vi "DataReplay.vi"() -> ()   [LabVIEW 2018]
uses:
  <vilib>/Waveform/WDTFileIO.llb/Read Waveform from File.vi
  <vilib>/measure/maspectr.llb/FFT Spectrum (Mag-Phase) for N Chan.vi
  <vilib>/Analysis/3filter.llb/Zero Phase Filter (DBL).vi
  <vilib>/Analysis/baseanly.llb/Inverse f Filter (DBL).vi
  <vilib>/Analysis/3filter.llb/FIR Windowed Filter (DBL).vi
  <vilib>/Analysis/NI_AALBase.lvlib
  <vilib>/measure/NI_MAPro.lvlib
panel:
  in  "CH2 历史数据 2":u32(ring) items=["矩形"=0, "Hanning"=1, "Hamming"=2, "Blackman"=5, "Flat Top"=6]
  out "第一次波形":bool=TRUE
  in  "滤波器类型":enum32{"零相位滤波器", "反幂律滤波器", "FIR滤波器", "中值滤波器"}(ring)
  in  "CH2 历史数据":u16(ring) items=["2021-07-14-11-34-43.csv"]
  in  "数据重置":bool
  in  "停止":bool
  in  "CH1 历史数据":u16(ring) items=["2021-07-14-11-34-43.csv"]
  out "频谱图":cluster{"f0":dbl, "df":dbl, "magnitude":dbl[]}[](graph)
  out "滤波":dynamicdata(graph)
  out "原波形":dynamicdata(graph)
  # "原波形"
  # "数据选择"
  # "滤波"
  # "频谱图"
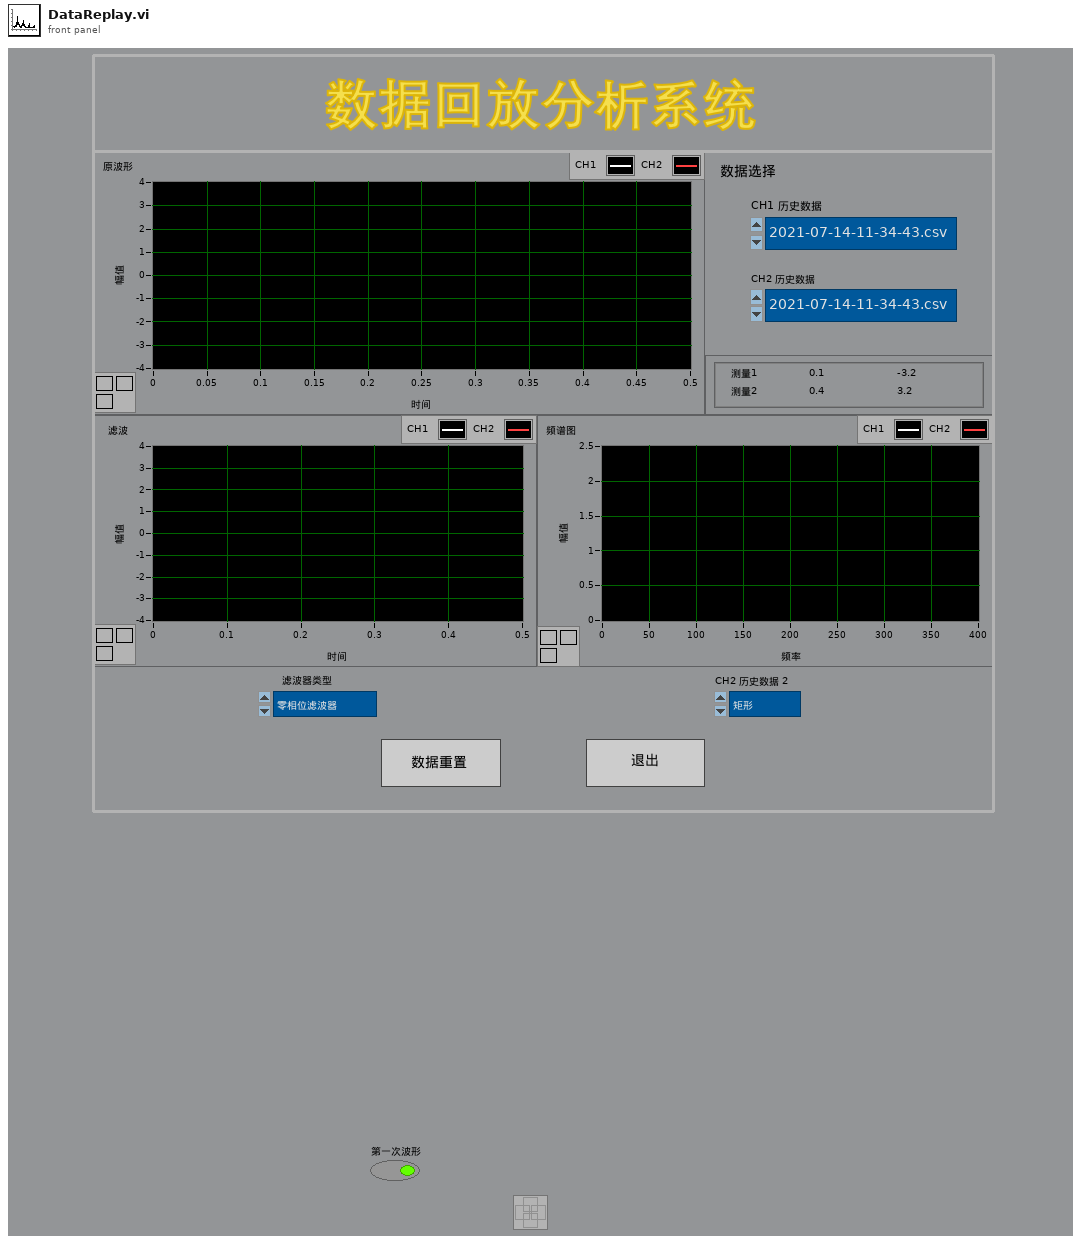
[diagram p1: front panel]
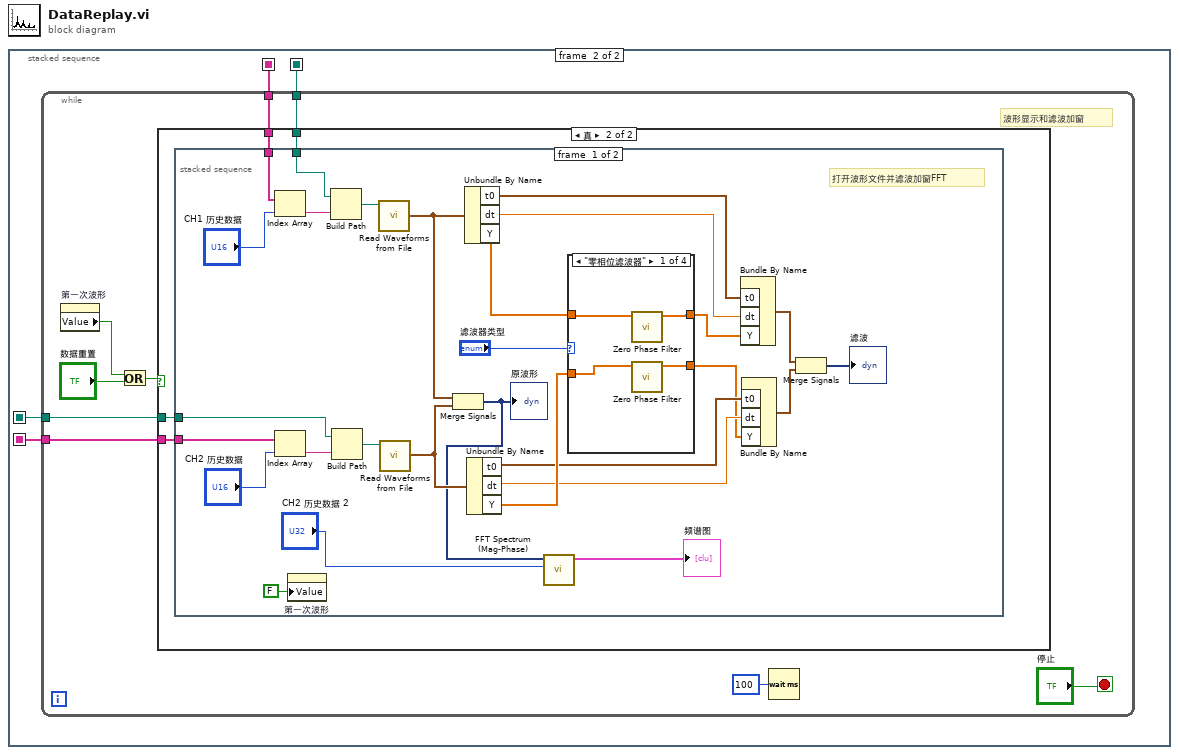
[diagram p0: block diagram]
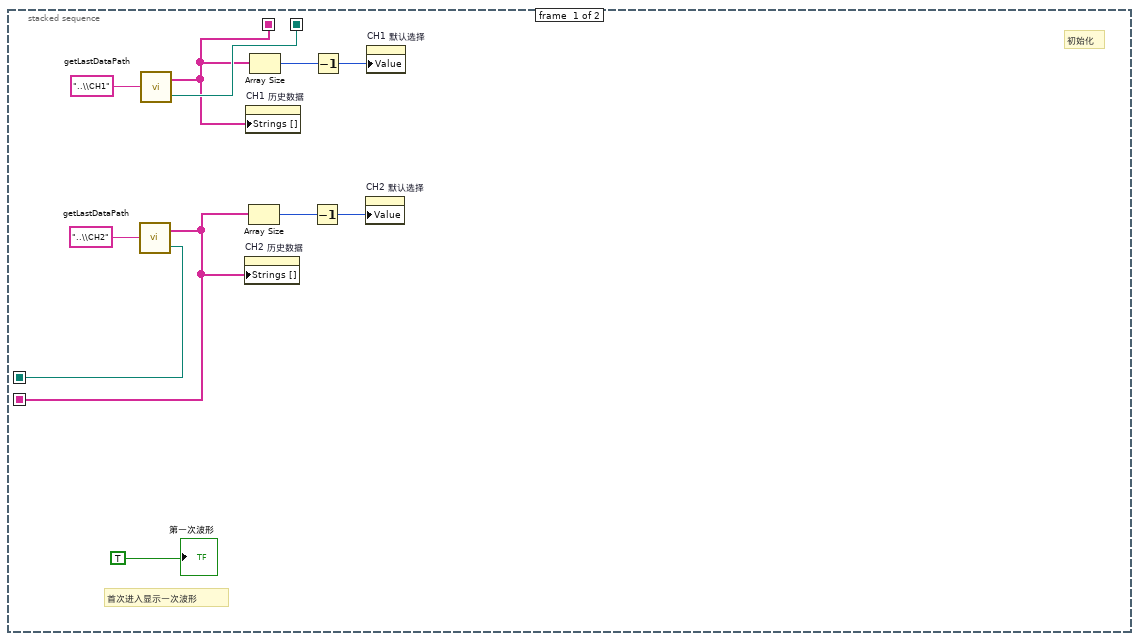
[diagram p2: hidden frame]
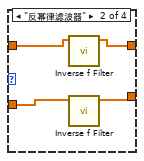
[diagram p4: hidden frame]
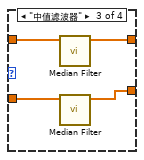
[diagram p5: hidden frame]
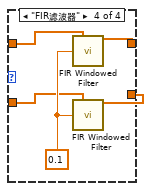
[diagram p6: hidden frame]
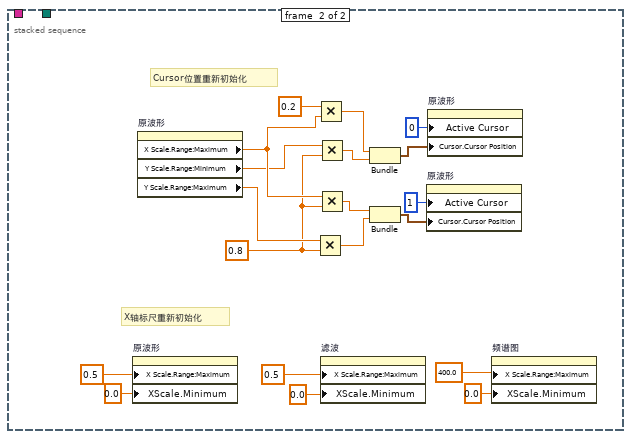
[diagram p7: hidden frame]
diagram:
  n1 = stacked-sequence {
    seq-local: [w8 _] -> [_ w15]
    seq-local: [w7 _] -> [_ w14]
    seq-local: [w2 _] -> [_ w12]
    seq-local: [w3 _] -> [_ w13]
    frame #0 {
      # "初始化"
      # "首次进入显示一次波形"
      n2 = call "getLastDataPath.vi"("文件夹输入"="..\\CH2" ("名称或相对路径")) -> ("数据文件名数组"=w2:string[], "文件夹路径"=w3:path)
      n3 = call "getLastDataPath.vi"("文件夹输入"="..\\CH1" ("名称或相对路径")) -> ("数据文件名数组"=w7:string[], "文件夹路径"=w8:path)
      n4 = property on="CH2 历史数据" class="Ring (严格)"("Strings []"=w2) -> ()  [unwired: 2 in, 2 out]
      n5 = property on="CH1 历史数据" class="Ring (严格)"("Strings []"=w7) -> ()  [unwired: 2 in, 2 out]
      n6 = Array Size(array=w2) -> (size(s)=w6:i32)
      n7 = Array Size(array=w7) -> (size(s)=w11:i32)
      n8 = Decrement(x=w6) -> (x-1=w5:i32)
      n9 = Decrement(x=w11) -> (x-1=w10:i32)
      n10 = property on="CH2 默认选择" class="Ring (严格)"("Value"=w5) -> ()  [unwired: 2 in, 2 out]
      n11 = property on="CH1 默认选择" class="Ring (严格)"("Value"=w10) -> ()  [unwired: 2 in, 2 out]
      "第一次波形" <- TRUE
    }
    frame #1 {
      n12 = while {
        tunnel: w15 -> [w22]
        tunnel: w14 -> [w21]
        tunnel: w13 -> [w20]
        tunnel: w12 -> [w19]
        stop <- "停止" stop-if-true
        # "波形显示和滤波加窗"
        n13 = property on="第一次波形" class="Bool (严格)"() -> ("Value"=w16:bool)  [unwired: 2 in, 2 out]
        n14 = Or(x=w16, y="数据重置") -> (x .or. y?=w17:bool)
        n15 = case shown="真" w17 {
          tunnel: w22 -> [_ w28]
          tunnel: w21 -> [_ w27]
          tunnel: w20 -> [_ w26]
          tunnel: w19 -> [_ w25]
          frame False {
          }
          frame True {
            n16 = stacked-sequence {
              tunnel: w28 -> [w53 _]
              tunnel: w27 -> [w52 _]
              tunnel: w26 -> [w48 _]
              tunnel: w25 -> [w47 _]
              frame #0 {
                # "打开波形文件并滤波加窗FFT"
                n17 = Index Array(array=w52, index="CH1 历史数据") -> (element=w55:string)
                n18 = Index Array(array=w47, index="CH2 历史数据") -> (element=w50:string)
                n19 = property on="第一次波形" class="Bool (严格)"("Value"=FALSE ("第一次波形")) -> ()  [unwired: 2 in, 2 out]
                n20 = Build Path(base path=w53, name or relative path=w55) -> (appended path=w54:path)
                n21 = Build Path(base path=w48, name or relative path=w50) -> (appended path=w49:path)
                n22 = call-poly <vilib>:"Read Waveforms from File.vi"("file path (dialog if empty)"=w54) -> ("first waveform in record"=w33:waveform(dbl))  [unwired: 5 in, 3 out]
                n23 = call-poly <vilib>:"Read Waveforms from File.vi"("file path (dialog if empty)"=w49) -> ("first waveform in record"=w32:waveform(dbl))  [unwired: 5 in, 3 out]
                n24 = Merge Signals(w33, w32) -> (w31:dynamicdata)
                "原波形" <- w31
                n25 = Unbundle By Name(w33) -> ("t0"=w42:timestamp, "dt"=w41:dbl, "Y"=w44:dbl[])
                n26 = Unbundle By Name(w32) -> ("t0"=w39:timestamp, "dt"=w38:dbl, "Y"=w43:dbl[])
                n27 = call-poly <vilib>:"FFT Spectrum (Mag-Phase).vi"("window"="CH2 历史数据 2", "time signals"=w31) -> ("magnitudes"=→"频谱图":cluster{"f0":dbl, "df":dbl, "magnitude":dbl[]}[])  [unwired: 5 in, 4 out]
                n28 = case shown="\"零相位滤波器\"" "滤波器类型" {
                  tunnel: w43 -> [w60 w64 w68 w72]
                  tunnel: [w59 w63 w67 w70] -> w40
                  tunnel: [w58 w62 w66 w71] -> w37
                  tunnel: w44 -> [w57 w61 w65 w69]
                  frame "零相位滤波器" {
                    n29 = call-poly <vilib>:"Zero Phase Filter.vi"("X"=w57) -> ("Filtered X"=w59:dbl[])  [unwired: 9 in, 1 out]
                    n30 = call-poly <vilib>:"Zero Phase Filter.vi"("X"=w60) -> ("Filtered X"=w58:dbl[])  [unwired: 9 in, 1 out]
                  }
                  frame "反幂律滤波器" {
                    n31 = call-poly <vilib>:"Inverse f Filter.vi"("X"=w61) -> ("Filtered X"=w63:dbl[])  [unwired: 6 in, 4 out]
                    n32 = call-poly <vilib>:"Inverse f Filter.vi"("X"=w64) -> ("Filtered X"=w62:dbl[])  [unwired: 6 in, 4 out]
                  }
                  frame "中值滤波器" {
                    n33 = call <vilib>:"Median Filter.vi"("X"=w65) -> ("Filtered X"=w67:dbl[])  [unwired: 9 in, 1 out]
                    n34 = call <vilib>:"Median Filter.vi"("X"=w68) -> ("Filtered X"=w66:dbl[])  [unwired: 9 in, 1 out]
                  }
                  frame "FIR滤波器" {
                    w73 = 0.1
                    n35 = call-poly <vilib>:"FIR Windowed Filter.vi"("X"=w69, "low cutoff freq: fl"=w73) -> ("Filtered X"=w70:dbl[])  [unwired: 12 in, 1 out]
                    n36 = call-poly <vilib>:"FIR Windowed Filter.vi"("X"=w72, "low cutoff freq: fl"=w73) -> ("Filtered X"=w71:dbl[])  [unwired: 12 in, 1 out]
                  }
                }
                n37 = Bundle By Name("t0"=w42, "dt"=w41, "Y"=w40) -> (w36:waveform(dbl))  [unwired: 1 in]
                n38 = Bundle By Name("t0"=w39, "dt"=w38, "Y"=w37) -> (w35:waveform(dbl))  [unwired: 1 in]
                n39 = Merge Signals(w36, w35) -> (→"滤波":dynamicdata)
              }
              frame #1 {
                w80 = 0.8 ("y")
                # "X轴标尺重新初始化"
                # "Cursor位置重新初始化"
                n40 = property on="原波形" class="WFGraph (严格)"("X Scale.Range:Maximum"=0.5 ("X标尺.范围:最大值"), "XScale.Minimum"=0.0 ("X标尺.范围:最小值")) -> ()  [unwired: 2 in, 2 out]
                n41 = property on="原波形" class="WFGraph (严格)"() -> ("X Scale.Range:Maximum"=w82:dbl, "Y Scale.Range:Minimum"=w81:dbl, "Y Scale.Range:Maximum"=w84:dbl)  [unwired: 2 in, 2 out]
                n42 = Multiply(x=w84, y=w80) -> (x*y=w85:dbl)
                n43 = Multiply(x=0.2, y=w82) -> (x*y=w88:dbl)
                n44 = Multiply(x=w81, y=w80) -> (x*y=w87:dbl)
                n45 = Multiply(x=w82, y=w80) -> (x*y=w83:dbl)
                n46 = property on="滤波" class="WFGraph (严格)"("X Scale.Range:Maximum"=0.5 ("X标尺.范围:最大值"), "XScale.Minimum"=0.0 ("X标尺.范围:最小值")) -> ()  [unwired: 2 in, 2 out]
                n47 = Bundle(w88, w87) -> (w92:cluster{dbl, dbl})  [unwired: 1 in]
                n48 = Bundle(w83, w85) -> (w89:cluster{dbl, dbl})  [unwired: 1 in]
                n49 = property on="原波形" class="WFGraph (严格)"("Active Cursor"=u32 1 ("活动游标"), "Cursor.Cursor Position"=w89) -> ()  [unwired: 2 in, 2 out]
                n50 = property on="原波形" class="WFGraph (严格)"("Active Cursor"=u32 0 ("活动游标"), "Cursor.Cursor Position"=w92) -> ()  [unwired: 2 in, 2 out]
                n51 = property on="频谱图" class="WFGraph (严格)"("X Scale.Range:Maximum"=400.0 ("X标尺.范围:最大值"), "XScale.Minimum"=0.0 ("X标尺.范围:最小值")) -> ()  [unwired: 2 in, 2 out]
              }
            }
          }
        }
        n52 = Wait (ms)(milliseconds to wait=u32 100 ("等待时间（毫秒）")) -> ()  [unwired: 1 out]
      }
    }
  }
